vi "Virtual Camera Start Live Mode.vi"(8 "error in (no error)":errorcluster, 10 "Camera Settings":T1={"Exposure Time (ms)"=100.0, "Binning"=enum."2x2", "Scan Mode (Flash)"=enum."Fast", "Trigger Mode (Flash)"=enum."Fast", "Frames to Acquire"=1000.0, "Pixel Correction (Flash)"=FALSE} {"Exposure Time (ms)" min=1.0 max=10000.0 step=1.0}, 11 "Virtual Camera in":refnum<class "Virtual Camera.lvclass">) -> (0 "error out":errorcluster, 3 "Virtual Camera out":refnum<class "Virtual Camera.lvclass">)   [LabVIEW 2018, in "Virtual Camera.lvlib" / "Virtual Camera.lvclass"]
uses:
  Virtual Camera.lvclass
  C:/Program Files/National Instruments/LabVIEW 2018/vi.lib/ActorFramework/Actor/Actor.lvclass
  Resources/Type Defs/Camera Settings.ctl
  Synchronization Device/Synchronization Device.lvclass
  Virtual Camera.lvclass/Virtual Camera.ctl
  Orca-Flash 4.0 V2 Messages/Flash Start Live Mode Msg/Flash Start Live Mode Msg.lvclass/Flash Start Live Mode Msg.ctl
  <vilib>/ActorFramework/Message Enqueuer/Message Enqueuer.lvclass/Message Enqueuer.ctl
  <vilib>/ActorFramework/Message Enqueuer/Enqueue.vi
  Orca-Flash 4.0 V2 Messages/Flash Start Live Mode Msg/Flash Start Live Mode Msg.lvclass
  C:/Program Files/National Instruments/LabVIEW 2018/vi.lib/ActorFramework/Message/Message.lvclass
  Resources/GLOBAL/GLOBAL Time-critical.vi
  <vilib>/ActorFramework/Message Priority Queue/Priority Enqueue.vi
  <vilib>/ActorFramework/Actor/Actor.lvclass
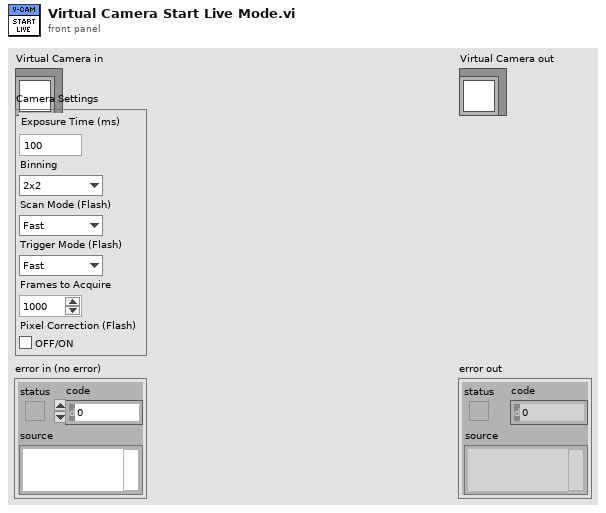
[diagram p1: front panel]
types:
  T1 = typedef "Camera Settings.ctl" = cluster{"Exposure Time (ms)":dbl, "Binning":enum16{"1x1", "2x2", "4x4"}, "Scan Mode (Flash)":enum16{"Fast", "Slow"}, "Trigger Mode (Flash)":enum16{"Fast", "Standard"}, "Frames to Acquire":dbl, "Pixel Correction (Flash)":bool}
  T2 = typedef "Semaphore RefNum" = refnum<k1>
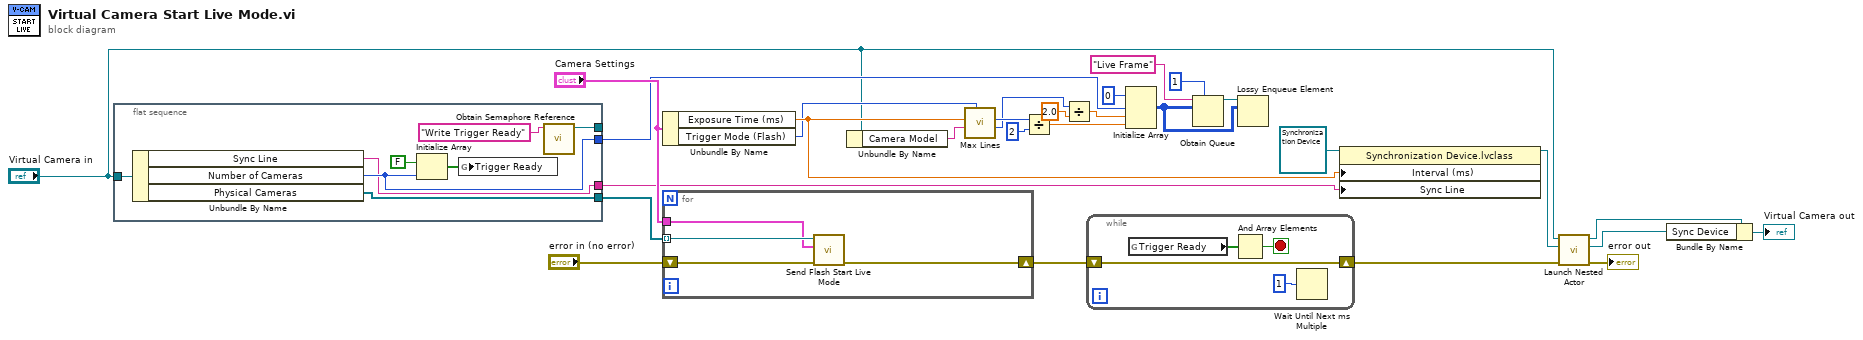
[diagram p0: block diagram]
diagram:
  n1 = flat-sequence {
    tunnel: [w36] -> w28
    tunnel: [w32] -> w23
    tunnel: "Virtual Camera in" -> [w35]
    tunnel: [w30] -> _
    tunnel: [w29] -> w6
    frame #0 {
      n2 = Unbundle By Name(w35) -> ("Sync Line"=w29:tag, "Number of Cameras"=w32:i32, "Physical Cameras"=w36:refnum<class "Message Enqueuer.lvclass">[])
      n3 = Initialize Array(FALSE, w32) -> (w33:bool[])
      n4 = global write "GLOBAL Time-critical.vi" "Trigger Ready"(w33) -> ()
      n5 = call <vilib>:"Obtain Semaphore Reference.vi"("name (unnamed)"="Write Trigger Ready") -> ("semaphore"=w30:T2)  [unwired: 4 in, 2 out]
    }
  }
  n6 = Unbundle By Name("Camera Settings") -> ("Exposure Time (ms)"=w12:dbl, "Trigger Mode (Flash)"=w11:enum16{"Fast", "Standard"})
  n7 = for {
    tunnel: w28 -> [w38] mode=indexing
    shift-right: [w39] -> w24
    shift-left: "error in (no error)" -> [w40]
    tunnel: "Camera Settings" -> [w37]
    n8 = call "Send Flash Start Live Mode.vi"("error in (no error)"=w40, "Camera Settings"=w37, "Message Enqueuer"=w38) -> ("error out"=w39:errorcluster)  [unwired: 7 in, 1 out]
  }
  n9 = Unbundle By Name("Virtual Camera in") -> ("Camera Model"=w1:string)
  n10 = call "Max Lines.vi"("Trigger Mode"=w11, "Camera Model"=w1, "Frame Time (ms)"=w12) -> ("upper limit"=w4:i32, "Max Lines"=w15:i32)  [unwired: 6 in, 1 out]
  n11 = Divide(x=w15, y=2) -> (x/y=w13:dbl)
  n12 = Divide(x=w4, y=2.0) -> (x/y=w5:dbl)
  n13 = while {
    shift-right: [w44] -> w20
    shift-left: w24 -> [w44]
    stop <- w42 stop-if-true
    n14 = global read "GLOBAL Time-critical.vi" "Trigger Ready"() -> (w43:bool[])
    n15 = And Array Elements(Boolean array=w43) -> (logical AND=w42:bool)
    n16 = Wait Until Next ms Multiple(millisecond multiple=u32 1) -> ()  [unwired: 1 out]
  }
  n17 = Initialize Array(u16 0, w23, w5, w13) -> (w7:u16[][][])
  n18 = Obtain Queue(max queue size (-1, unlimited)=1, name (unnamed)="Live Frame", element data type=w7) -> (queue out=w8:refnum<queue>)  [unwired: 2 in, 2 out]
  n19 = Lossy Enqueue Element(queue=w8, element=w7) -> ()  [unwired: 1 in, 4 out]
  n20 = property class="Synchronization Device.lvclass"(reference=refnum<class "Synchronization Device.lvclass"> refnum ("Synchronization Device.lvlib:Synchronization Device.lvclass"), "Interval (ms)"=w12, "Sync Line"=w6) -> (reference out=w21:refnum<class "Synchronization Device.lvclass">)  [unwired: 1 in, 1 out]
  n21 = call <vilib>:"Launch Nested Actor.vi"("error in (no error)"=w20, "Nested Actor"=w21, "Caller Actor in"="Virtual Camera in") -> ("error out"=→"error out":errorcluster, "Nested Actor's Enqueuer"=w16:refnum<class "Message Enqueuer.lvclass">, "Caller Actor out"=w18:refnum<class "Virtual Camera.lvclass">)  [unwired: 6 in]
  n22 = Bundle By Name(cluster=w18, "Sync Device"=w16) -> (→"Virtual Camera out":refnum<class "Virtual Camera.lvclass">)
